vi "reg-log-ntr.vi"(6 "Operation(Read)":T3, 8 "error in":errorcluster, 10 "filter by proc name":cluster{"ProcName":string, "StepIndex":i32}={"ProcName"="", "StepIndex"=-1}, 11 "Reports to Collect":T4 {"clk" format="%#.3f"}) -> (0 "error out":errorcluster, 2 "compact report":T1[](array[typedef]) {"clk" format="%#.1f"}, 3 "Collected Reports":T4[](array[typedef]) {"clk" format="%#.3f"})   [LabVIEW 2024]
uses:
  controls/typeEngineLogCluster.ctl
  controls/type.StepFunction.ctl
  controls/enum.report-filter.ctl
  controls/UiCompactReport.ctl
panel:
  out "size(s)":i32
  in  "Rows":i32=20
  # "stepIndex>=0 then filter by step index\nstepIndex==-1 then do not filter"
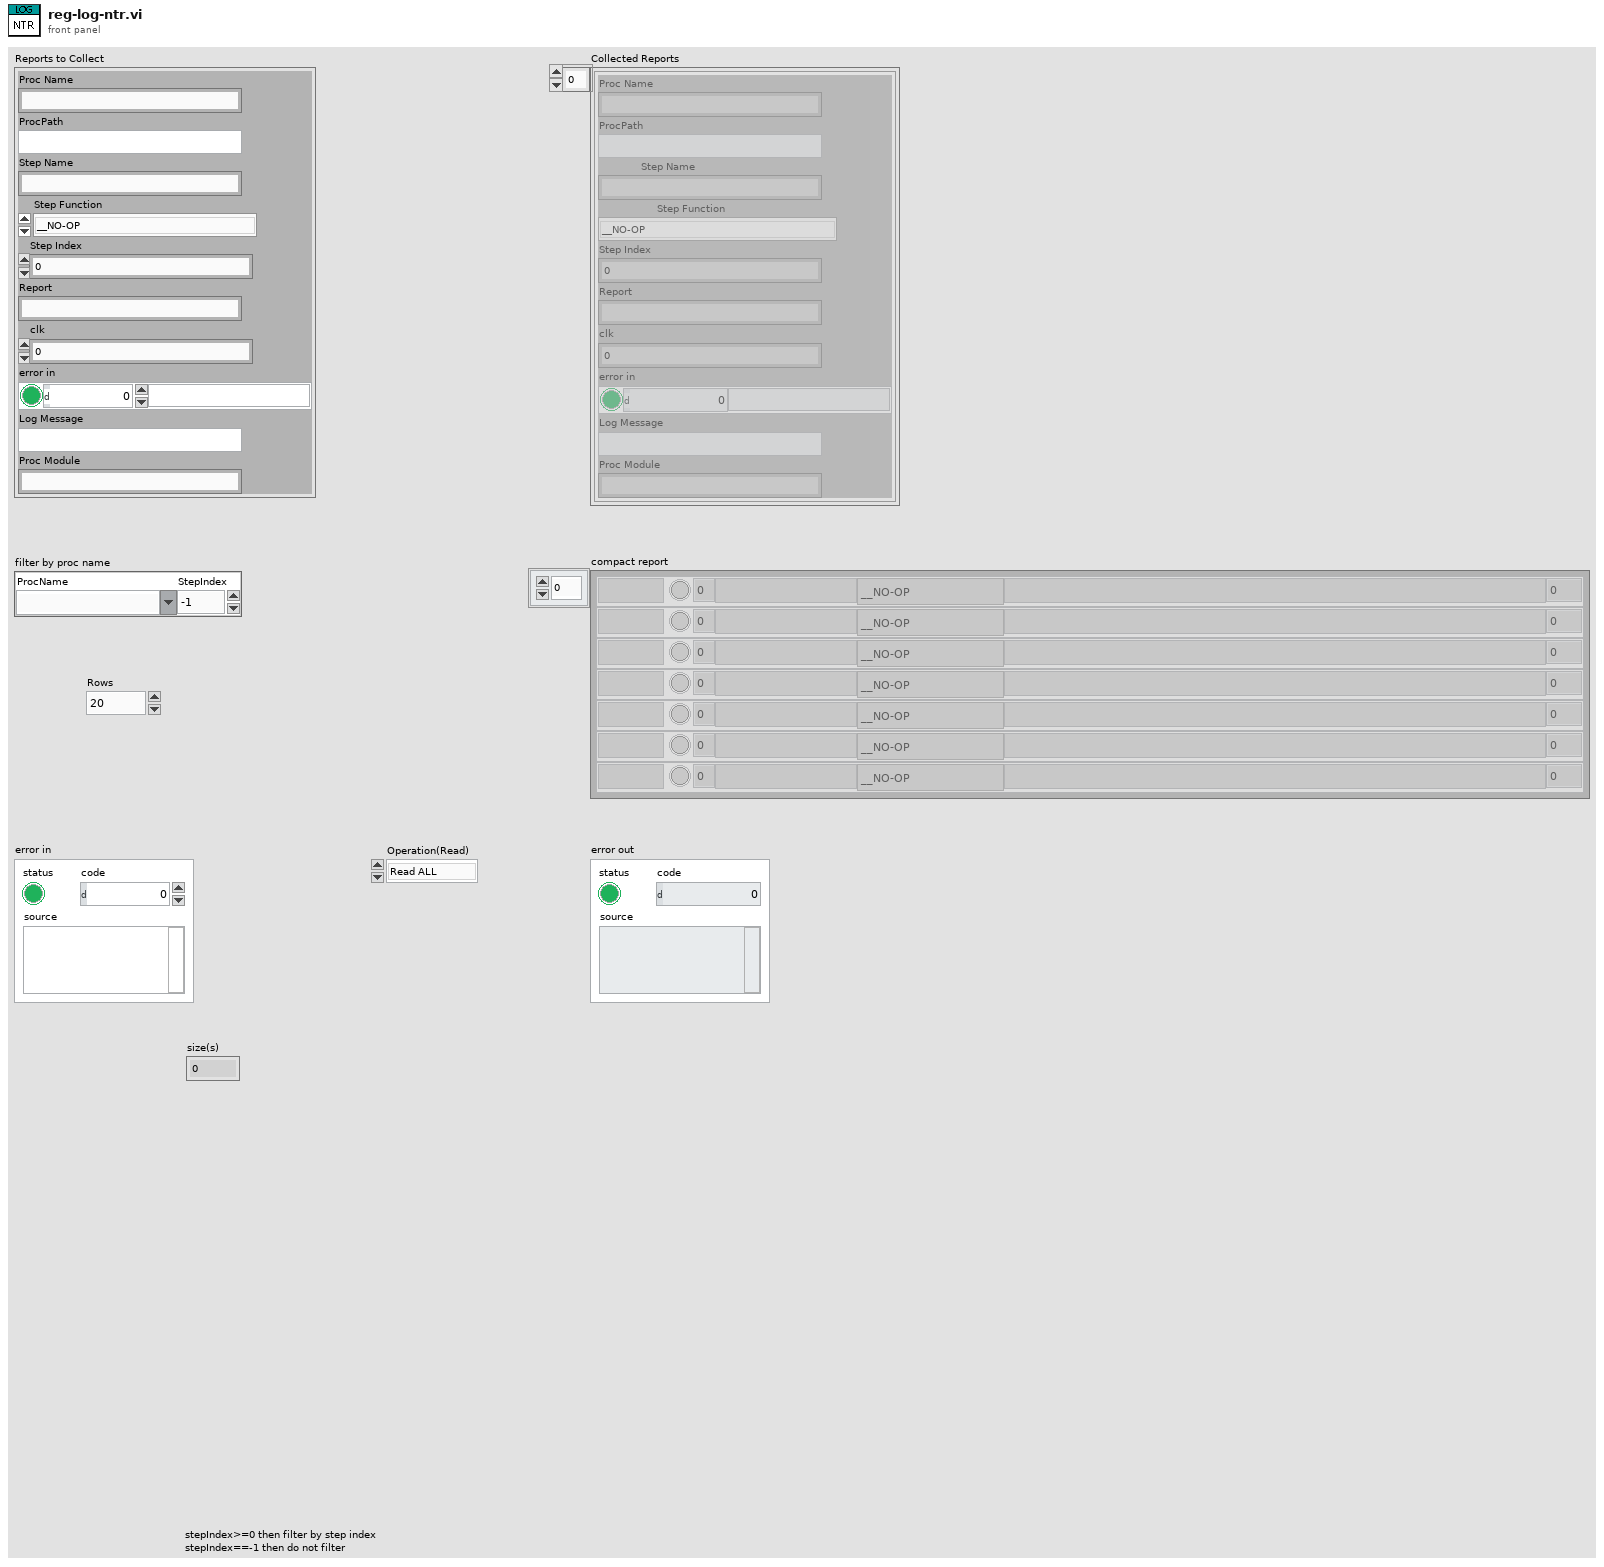
[diagram p1: front panel]
types:
  T1 = typedef "UiCompactReport.ctl" = cluster{"ErrorFlag":bool, "idx":i32, "Step Name":string, "Step Function":T2, "Report":string, "clk":dbl, "Proc":string}
  T2 = typedef "type.StepFunction.ctl" = enum16{"__NO-OP", "_DELAY_LOAD", "_DELAY_COMPARE", "_JUMP", "_COMPLETE", "_COMPARE", "_LOG_MESSAGE", "_LOG_LAST_REPORT", "_SCHEDULE", "_SCHED_DAILY", "CLK_COMPARE", "PROC_START", "PROC_STOP", "PROC_LOAD", "PROC_COMPLETION_CHECK", "PROC_COMPLETION_LOAD", "_IO_READ", "_IO_READ_MANY", "_IO_WRITE", "_IO_WRITE_BY_REG", "_IO_GET_OUTPUT", "_OCS_CHECK", "_OCS_RECORD", "_GET_RH", "_GET_ACC_UV", "_GET_WD", "_GET_WS", "_REC_DELETE", "_REC_MOVE", "_REC_COPY", "_IRR_CHECK", "UNIT_CHECK", "UNIT_SAMPLE", "UNIT_DOSE"}
  T3 = typedef "enum.report-filter.ctl" = enum16{"Read ALL", "Read Errors", "Collect", "ClearAll"}
  T4 = typedef "typeEngineLogCluster.ctl" = cluster{"Proc Name":string, "ProcPath":string, "Step Name":string, "Step Function":T2, "Step Index":i32, "Report":string, "clk":dbl, "error in":errorcluster, "Log Message":string, "Proc Module":string}
  T5 = cluster{"Proc Name":bool, "ProcPath":bool, "Step Name":bool, "Step Function":bool, "Step Index":bool, "Report":bool, "clk":bool, "error in":cluster{"status":bool, "code":bool, "source":bool}, "Log Message":bool, "Proc Module":bool}
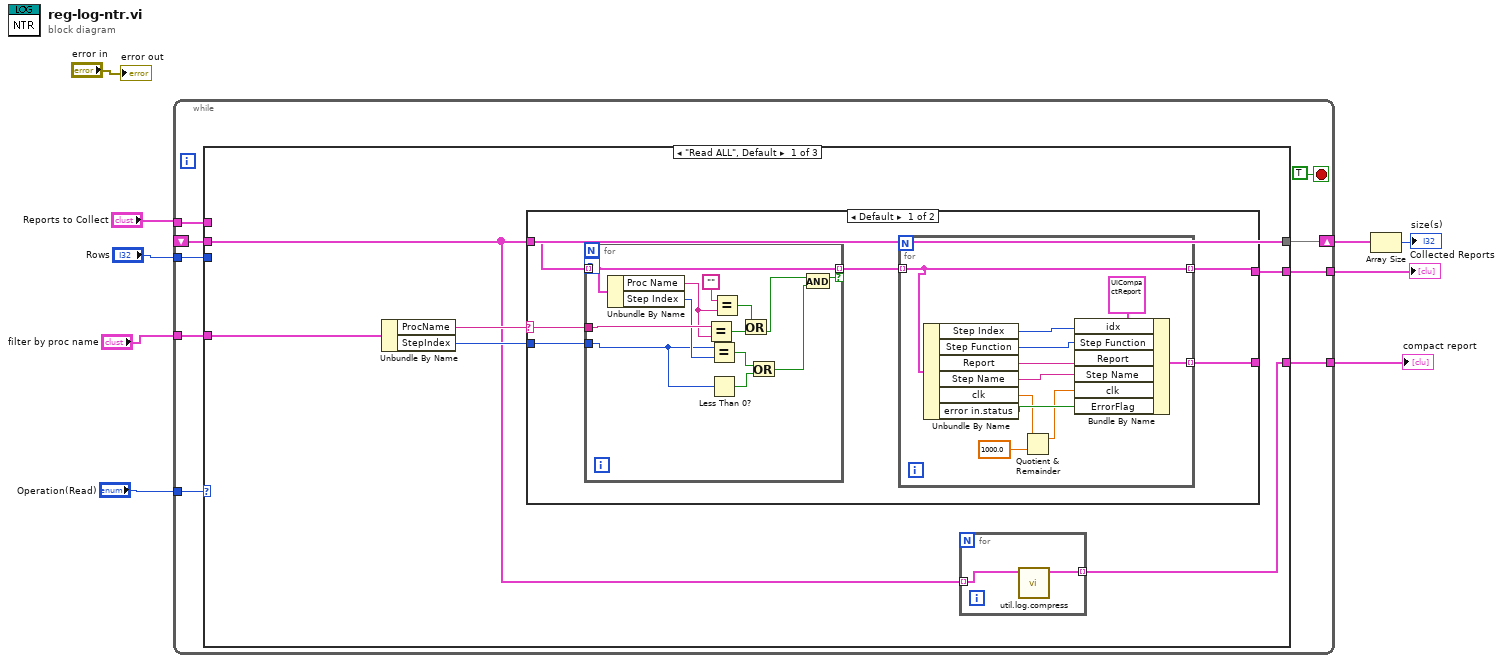
[diagram p0: block diagram]
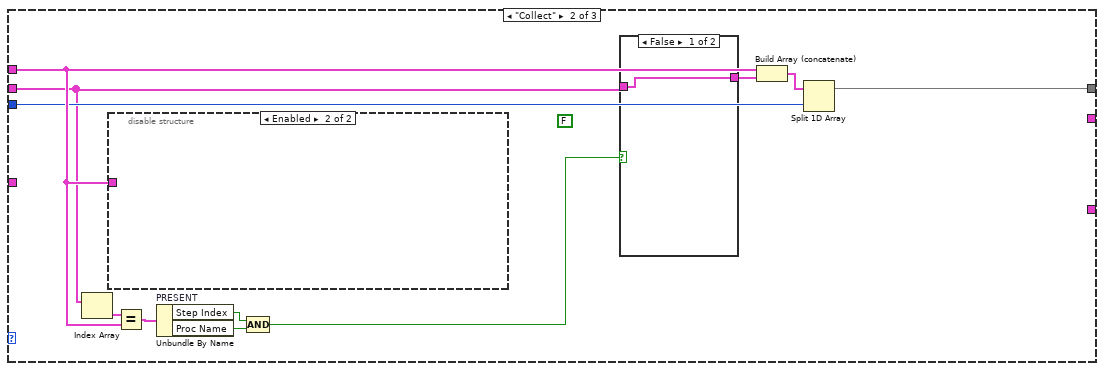
[diagram p3: hidden frame]
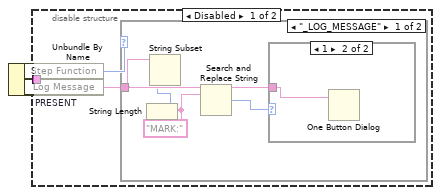
[diagram p4: hidden frame]
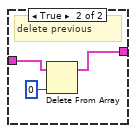
[diagram p7: hidden frame]
diagram:
  n1 = while {
    shift-right: [w16] -> w6
    shift-left: _ -> [w14]
    tunnel: "Reports to Collect" -> [w18]
    tunnel: "Rows" -> [w15]
    tunnel: "Operation(Read)" -> [w13]
    tunnel: [w12] -> w4
    tunnel: [w11] -> w3
    tunnel: "filter by proc name" -> [w10]
    stop <- TRUE stop-if-true
    n2 = case shown="\"Read ALL\", Default" w13 {
      tunnel: w18 -> [_ w68 _]
      tunnel: [w20 w67 _] -> w16
      tunnel: w15 -> [_ w66 _]
      tunnel: w14 -> [w20 w65 _]
      tunnel: [w24 _ _] -> w12
      tunnel: [w19 _ _] -> w11
      tunnel: w10 -> [w21 _ _]
      frame "Read ALL", Default {
        n3 = Unbundle By Name(w21) -> ("ProcName"=w23:string, "StepIndex"=w22:i32)
        n4 = case shown="Default" w23 {
          selector: w23 -> [w31 _]
          tunnel: w20 -> [w32 w57]
          tunnel: [w28 w57] -> w24
          tunnel: w22 -> [w30 _]
          tunnel: [w27 _] -> _
          frame Default {
            n5 = for {
              tunnel: w32 -> [w44] mode=indexing
              tunnel: w31 -> [w55]
              tunnel: [w44] -> w29 mode=indexing if=w50
              tunnel: w30 -> [w53]
              workers-P: _ -> [_]
              n6 = Unbundle By Name(w44) -> ("Proc Name"=w47:string, "Step Index"=w54:i32)
              n7 = Equal?(x=w55, y=w47) -> (x = y?=w56:bool)
              n8 = Equal?(x=w53, y=w54) -> (x = y?=w52:bool)
              n9 = Less Than 0?(x=w53) -> (x < 0?=w51:bool)
              n10 = Equal?(x="", y=w47) -> (x = y?=w45:bool)
              n11 = Or(x=w45, y=w56) -> (x .or. y?=w48:bool)
              n12 = Or(x=w52, y=w51) -> (x .or. y?=w49:bool)
              n13 = And(x=w48, y=w49) -> (x .and. y?=w50:bool)
            }
            n14 = for {
              tunnel: w29 -> [w42] mode=indexing
              tunnel: [w42] -> w28 mode=indexing
              tunnel: [w43] -> w27 mode=indexing
              n15 = Unbundle By Name(w42) -> ("Step Index"=w38:i32, "Step Function"=w37:T2, "Report"=w40:string, "Step Name"=w39:string, "clk"=w35:dbl, "error in.status"=w36:bool)
              n16 = Quotient & Remainder(x=w35, y=1000.0) -> (x-y*floor(x/y)=w33:dbl)  [unwired: 1 out]
              n17 = Bundle By Name(cluster=T1 {"ErrorFlag"=FALSE, "idx"=0, "Step Name"="", "Step Function"=enum."__NO-OP", "Report"="", "clk"=0.0, "Proc"=""} ("compact report 2"), "idx"=w38, "Step Function"=w37, "Report"=w40, "Step Name"=w39, "clk"=w33, "ErrorFlag"=w36) -> (w43:T1)
            }
          }
          frame "" {
          }
        }
        n18 = for {
          tunnel: w20 -> [w25] mode=indexing
          tunnel: [w26] -> w19 mode=indexing
          n19 = call "util.log.compress.vi"("Log Cluster in"=w25) -> ("Compact Report"=w26:T1)  [unwired: 9 in, 1 out]
        }
      }
      frame "Collect" {
        (unwired) FALSE
        n20 = Index Array(array=w65) -> (element=w58:T4)  [unwired: 1 in]
        n21 = disable-structure shown="Enabled" {
          disable-tunnel: w68 -> [w71 _]
          frame Disabled {
            n22 = Unbundle By Name "PRESENT"(w71) -> ("Step Function"=w69:T2, "Log Message"=w70:string)
            n23 = case shown="\"_LOG_MESSAGE\"" w69 {
              tunnel: w70 -> [w75 _]
              frame "_LOG_MESSAGE" {
                w73 = "MARK:" ("search string")
                n24 = String Length(string=w73) -> (length=w74:i32)
                n25 = String Subset(string=w75, length (rest)=w74) -> ()  [unwired: 1 in, 1 out]
                n26 = Search and Replace String(input string=w75, search string=w73) -> (result string=w72:string, number of replacements=w76:i32)  [unwired: 6 in, 2 out]
                n27 = case shown="1" w76 {
                  tunnel: w72 -> [_ w77]
                  frame 0, Default {
                  }
                  frame 1 {
                    n28 = One Button Dialog(message=w77) -> ()  [unwired: 1 in, 1 out]
                  }
                }
              }
              frame Default {
              }
            }
          }
          frame Enabled {
          }
        }
        n29 = Equal?(x=w58, y=w68) -> (x = y?=w61:T5)
        n30 = Unbundle By Name "PRESENT"(w61) -> ("Step Index"=w59:bool, "Proc Name"=w60:bool)
        n31 = Compound Arithmetic op=AND(w59, w60) -> (w62:bool)
        n32 = case shown="False" w62 {
          tunnel: w65 -> [w78 w81]
          tunnel: [w78 w80] -> w64
          frame False {
          }
          frame True {
            # "delete previous"
            n33 = Delete From Array(array=w81, index=0) -> (array with subset deleted=w80:T4[])  [unwired: 1 in, 1 out]
          }
        }
        n34 = Build Array (concatenate)(w68, w64) -> (w63:T4[])
        n35 = Split 1D Array(array=w63, index=w66) -> (first subarray=w67:T4[])  [unwired: 1 out]
      }
      frame "ClearAll" {
      }
    }
  }
  "Collected Reports" <- w4
  "compact report" <- w3
  n36 = Array Size(array=w6) -> (size(s)=→"size(s)":i32)
  "error out" <- "error in"
